vi "DumbDash Find Controls.vi"(11 "ControlsOnPage":refnum<vi>[](array[refnum])) -> (3 "Found Controls":refnum<vi>[](array[refnum]))   [LabVIEW 2014]
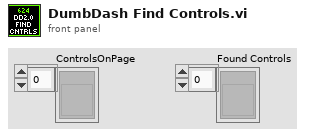
[diagram p1: front panel]
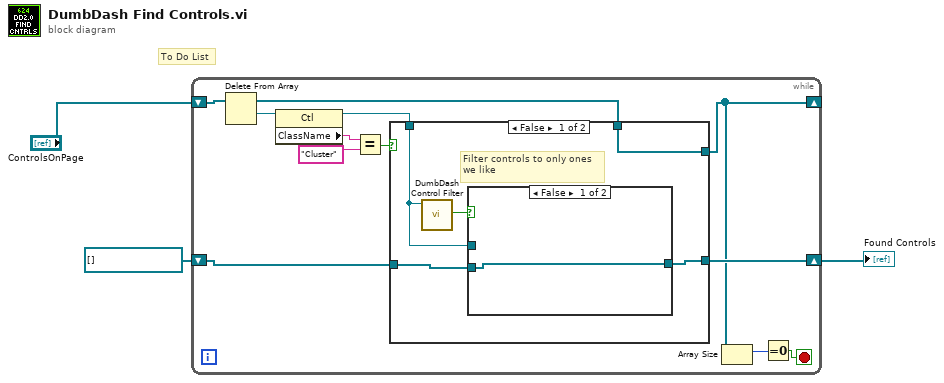
[diagram p0: block diagram]
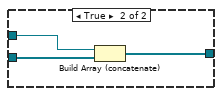
[diagram p2: hidden frame]
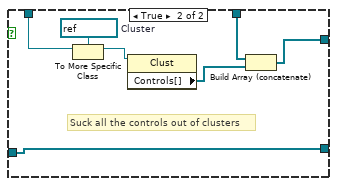
[diagram p3: hidden frame]
diagram:
  # "To Do List"
  n1 = while {
    shift-right: [w6] -> _
    shift-left: "ControlsOnPage" -> [w13]
    shift-right: [w8] -> w1
    shift-left: refnum<vi>[] [] -> [w7]
    stop <- w4 stop-if-true
    n2 = Delete From Array(array=w13) -> (deleted portion=w12:refnum<vi>, array with subset deleted=w9:refnum<vi>[])  [unwired: 2 in]
    n3 = property class="Ctl"(reference=w12) -> (reference out=w10:refnum<vi>, "ClassName"=w15:string)  [unwired: 1 in, 1 out]
    n4 = Equal?(x=w15, y="Cluster") -> (x = y?=w11:bool)
    n5 = case shown="False" w11 {
      tunnel: w10 -> [w17 w31]
      tunnel: w9 -> [w20 w28]
      tunnel: [w20 w26] -> w6
      tunnel: [w19 w25] -> w8
      tunnel: w7 -> [w18 w25]
      frame False {
        # "Filter controls to only ones\nwe like"
        n6 = call "DumbDash Control Filter.vi"("Ctl Refnum"=w17) -> ("Keep?"=w16:bool)  [unwired: 10 in]
        n7 = case shown="False" w16 {
          tunnel: w17 -> [_ w24]
          tunnel: [w21 w23] -> w19
          tunnel: w18 -> [w21 w22]
          frame False {
          }
          frame True {
            n8 = Build Array (concatenate)(w24, w22) -> (w23:refnum<vi>[])
          }
        }
      }
      frame True {
        w30 = refnum<vi> refnum  # Cluster
        # "Suck all the controls out of clusters"
        n9 = To More Specific Class(target class=w30, reference=w31) -> (specific class reference=w29:refnum<vi>)  [unwired: 1 in, 1 out]
        n10 = property class="Clust"(reference=w29) -> ("Controls[]"=w27:refnum<vi>[])  [unwired: 1 in, 2 out]
        n11 = Build Array (concatenate)(w28, w27) -> (w26:refnum<vi>[])
      }
    }
    n12 = Array Size(array=w6) -> (size(s)=w5:i32)
    n13 = Equal To 0?(x=w5) -> (x = 0?=w4:bool)
  }
  "Found Controls" <- w1
